vi "SVA 4MV6 T027 CCE.vi"(7 "NORMALIZACIÓN":bool, 9 "UMBRAL":u8(knob) scale=0.0..255.0, 10 "CAPA DE COLOR":T1(ring), 11 "RUTA DE IMAGEN":path) -> (2 "MOMENTOS INVARIANTES DE HU":dbl[](array[numeric]), 3 "IMAGEN BINARIZADA":picture)   [LabVIEW 2020]
panel:
  in  "INVERTIDO?":bool
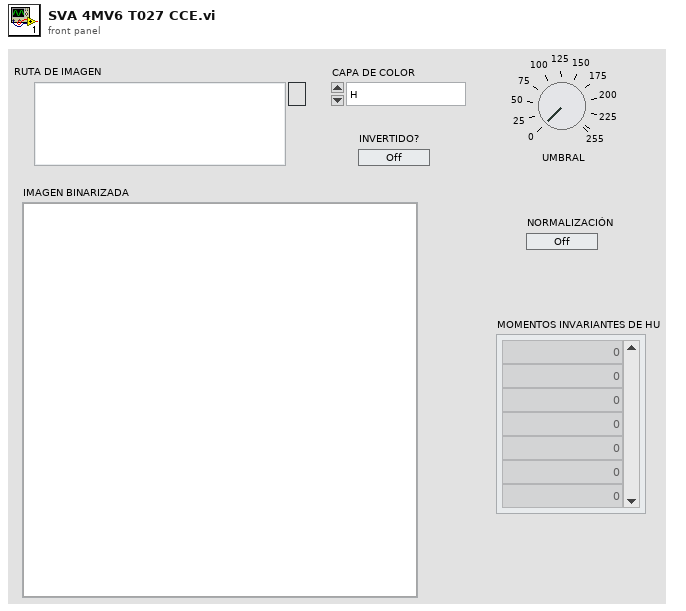
[diagram p1: front panel]
types:
  T1 = enum16{"H", "S", "V", "C", "M", "Y", "R", "G", "B", "RGB2GRAY MATLAB"}
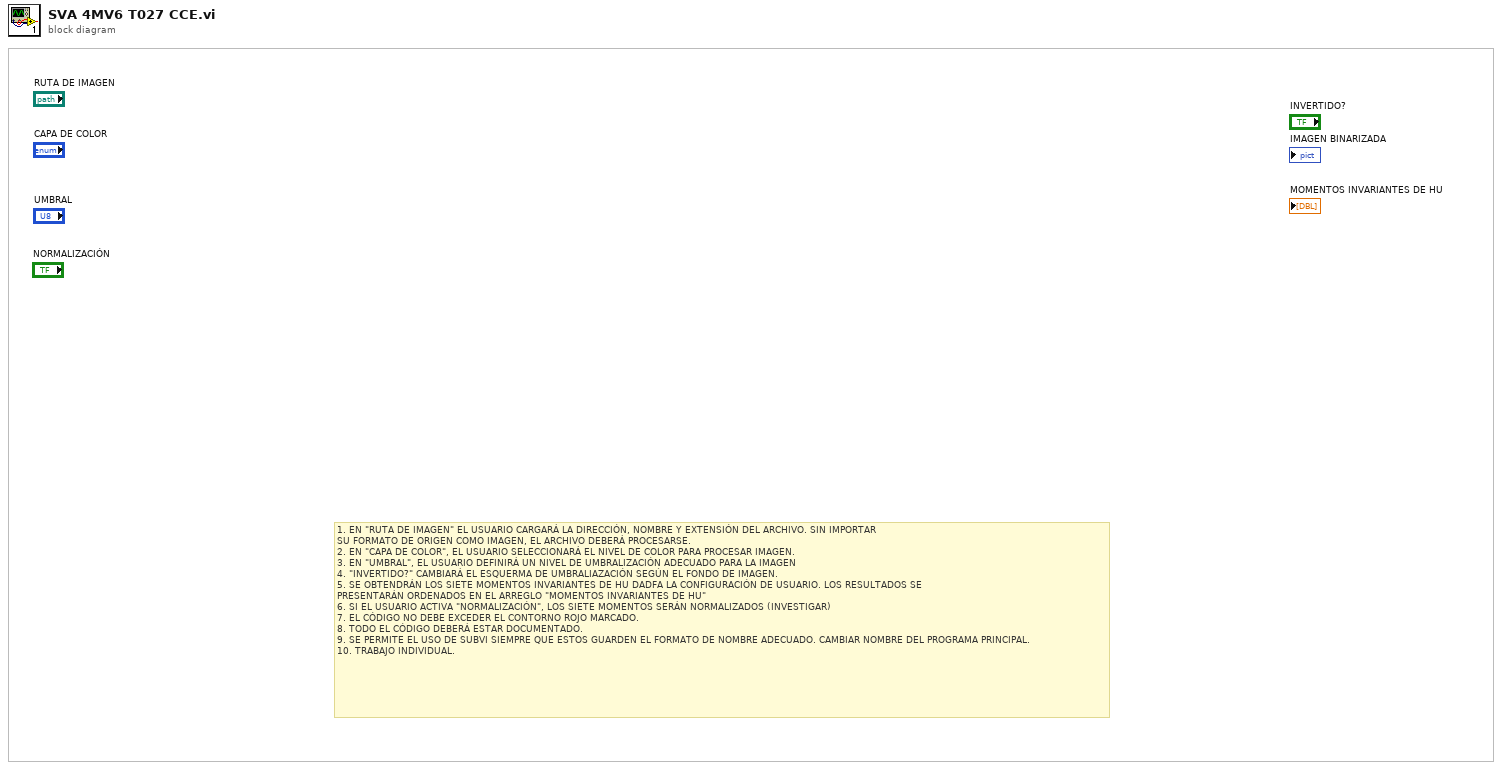
[diagram p0: block diagram]
diagram:
  # "1. EN \"RUTA DE IMAGEN\" EL USUARIO CARGARÁ LA DIRECCIÓN, NOMBRE Y EXTENSIÓN DEL ARCHIVO. SIN IMPORTAR \nSU FORMATO DE ORIGEN COMO IMAGEN, EL ARCHIVO DEBERÁ PROCESARSE. \n2. EN \"CAPA DE COLOR\", EL USUARIO SELECCIONARÁ EL NIVEL DE COLOR PARA PROCESAR IMAGEN. \n3. EN \"UMBRAL\", EL USUARIO DEFINIRÁ UN NIVEL DE UMBRALIZACIÓN ADECUADO PARA LA IMAGEN \n4. \"INVERTIDO?\" CAMBIARÁ EL ESQUERMA DE UMBRALIAZACIÓN SEGÚN EL FONDO DE IMAGEN. \n5. SE OBTENDRÁN LOS SIETE MOMENTOS INVARIANTES DE HU DADFA LA CONFIGURACIÓN DE USUARIO. LOS RESULTADOS SE \nPRESENTARÁN ORDENADOS EN EL ARREGLO \"MOMENTOS INVARIANTES DE HU\"\n6. SI EL USUARIO ACTIVA \"NORMALIZACIÓN\", LOS SIETE MOMENTOS SERÁN NORMALIZADOS (INVESTIGAR) \n7. EL CÓDIGO NO DEBE EXCEDER EL CONTORNO ROJO MARCADO. \n8. TODO EL CÓDIGO DEBERÁ ESTAR DOCUMENTADO. \n9. SE PERMITE EL USO DE SUBVI SIEMPRE QUE ESTOS GUARDEN EL FORMATO DE NOMBRE ADECUADO. CAMBIAR NOMBRE DEL PROGRAMA PRINCIPAL. \n10. TRABAJO INDIVIDUAL."
